vi "TL4000 Switch TEC Output.vi"(8 "error in (no error)":errorcluster {"code" format="%.0x"}, 10 "TEC Output (Off)":bool, 11 "instrument handle":refnum<visa-resource-name>) -> (0 "error out":errorcluster {"code" format="%.0x"}, 3 "instrument handle out":refnum<visa-resource-name>)   [LabVIEW 2019]
doc: "This VI switches the TEC output on/off.\n\nNote: \nThis VI is valid for: TED4000, ITC4000, CLD1000"
uses:
  TL4000_32.dll
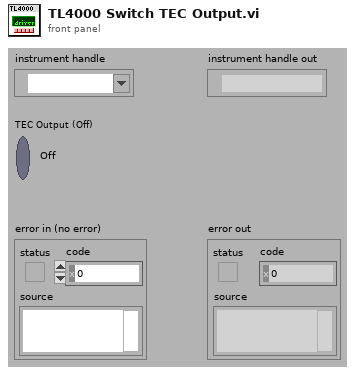
[diagram p1: front panel]
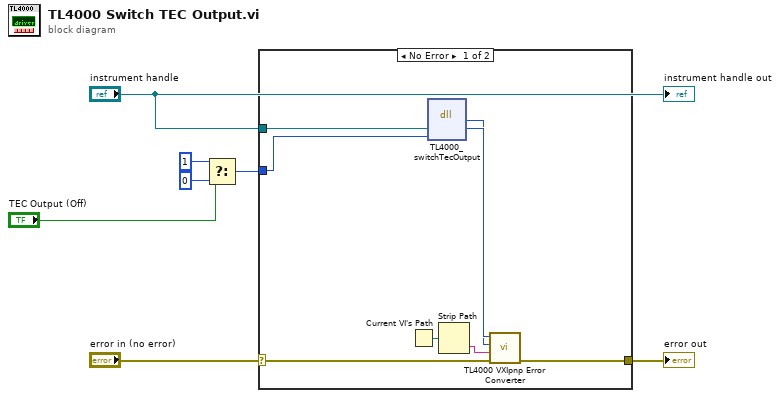
[diagram p0: block diagram]
diagram:
  n1 = Select(t=u16 1, s="TEC Output (Off)", f=u16 0) -> (s? t:f=w1:u16)
  n2 = case shown="No Error" "error in (no error)" {
    selector: "error in (no error)" -> [w10 w16]
    tunnel: [w9 w16] -> w7
    tunnel: "instrument handle" -> [w14 _]
    tunnel: w1 -> [w8 _]
    frame No Error {
      n3 = Current VI's Path() -> (path=w15:path)
      n4 = dll-call lib="TL4000_32.*" fn="TL4000_switchTecOutput"("Instrument Handle"=w14, "TEC Output"=w8) -> (w12:i32, "Instrument Handle"=w13:u32)  [unwired: 4 in, 2 out]
      n5 = Strip Path(path=w15) -> (name=w11:string)  [unwired: 1 out]
      n6 = call "TL4000 VXIpnp Error Converter.vi"("error in (no error)"=w10, "Name Of VI (\"\")"=w11, "CVI Error Code (0)"=w12, "instrument handle"=w13) -> ("error out"=w9:errorcluster)  [unwired: 6 in, 1 out]
    }
    frame Error {
    }
  }
  "error out" <- w7
  "instrument handle out" <- "instrument handle"
